vi "DAQ.vi"(0 "Queues":T1, 3 "error in (no error)":errorcluster) -> (10 "error out":errorcluster)   [LabVIEW 2014]
uses:
  CMD UI enum.ctl
  CMD Report enum.ctl
  CMD DA enum.ctl
  CMD DAQ enum.ctl
  CMD LOG enum.ctl
  set_get.ctl
  patiant and daq params.ctl
  <vilib>/DAQmx/create/channels.llb/DAQmx Create Channel (AI-Voltage-Basic).vi
  <vilib>/DAQmx/configure/timing.llb/DAQmx Timing (Sample Clock).vi
  <vilib>/DAQmx/read.llb/DAQmx Read (Analog 2D DBL NChan NSamp).vi
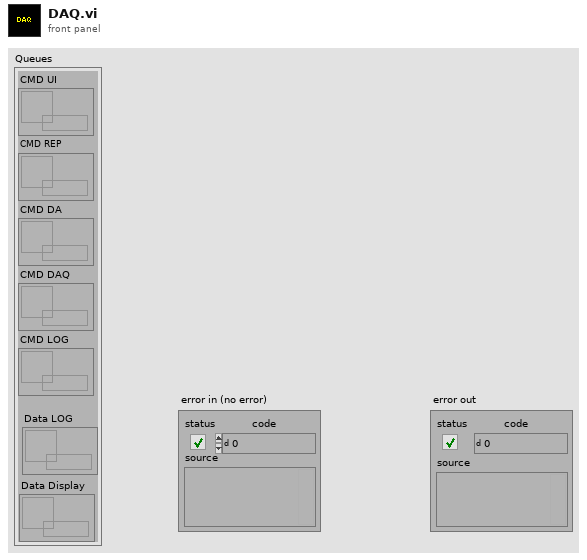
[diagram p1: front panel]
types:
  T1 = cluster{"CMD UI":refnum<queue>, "CMD REP":refnum<queue>, "CMD DA":refnum<queue>, "CMD DAQ":refnum<queue>, "CMD LOG":refnum<queue>, "Data LOG":refnum<queue>, "Data Display":refnum<queue>}
  T2 = typedef "patiant and daq params.ctl" = cluster{"DAQ Parameters":cluster{"Sampling rate":dbl, "Max_volt":dbl, "Min_volt":dbl, "DAQmx Physical Channels \nHR,SC":tag, "Resting State":bool, "Analyze every (s)":dbl}, "Patient Info \n(Updates automatically when reading from file)":cluster{"Patient Name":string, "Patient ID":string, "Patient Age":dbl, "Gender":string}, "Raw Data Read Path":path, "Avg HR ":dbl, "Avg SC  ":dbl}
  T3 = typedef "CMD DAQ enum.ctl" = enum16{"Init DAQ", "Init Read From File", "DAQ", "Read From File", "Stop DAQ", "Stop Read From File", "Exit"}
  T4 = typedef "set_get.ctl" = enum16{"Set", "Get"}
  T5 = typedef "CMD UI enum.ctl" = enum16{"Init all", "Update Patient Info", "Update Analyzed", "Create Report", "Analyze Data", "Start DAQ", "Start Read", "LOG Data", "Stop LOG Data", "Stop DAQ", "Stop Read", "EXIT"}
  T6 = enum16{"open", "replace", "create", "open or create", "replace or create", "replace or create with confirmation"}
  T7 = cluster{string, string, dbl, "Combo Box":string, dbl}
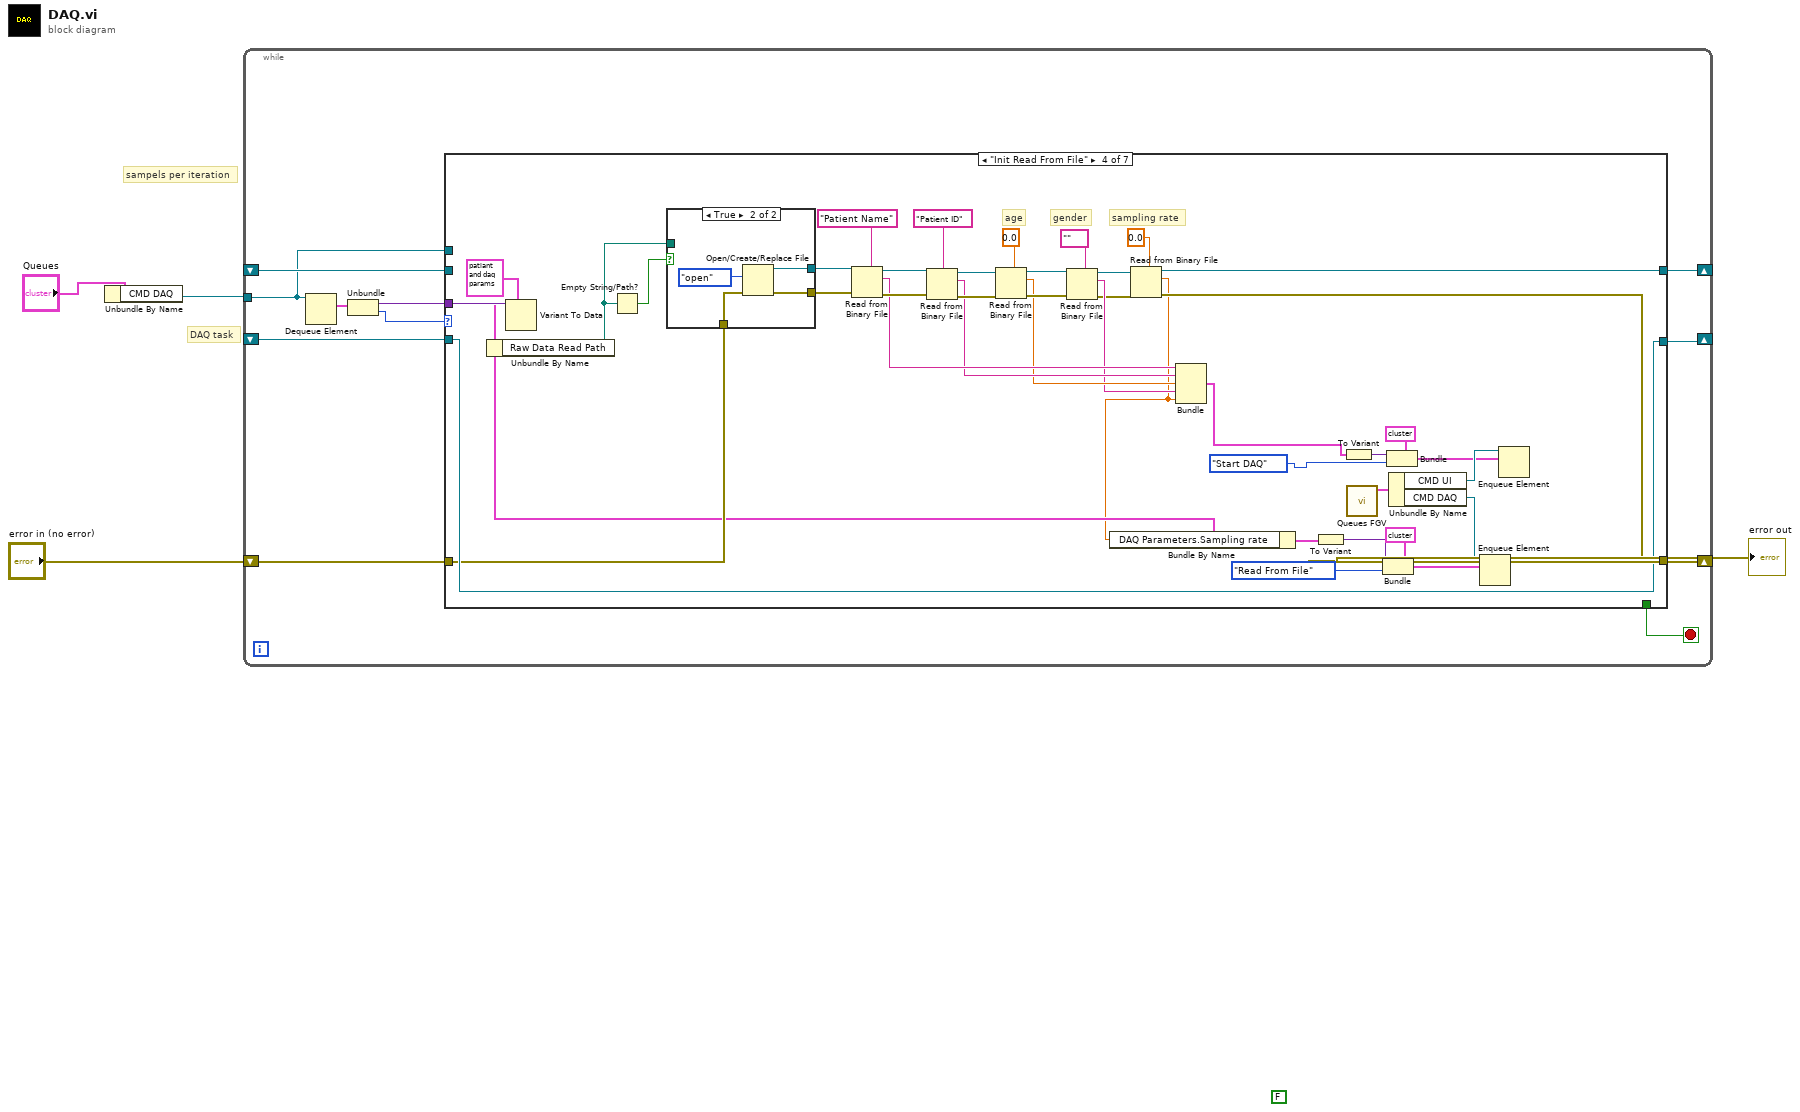
[diagram p0: block diagram]
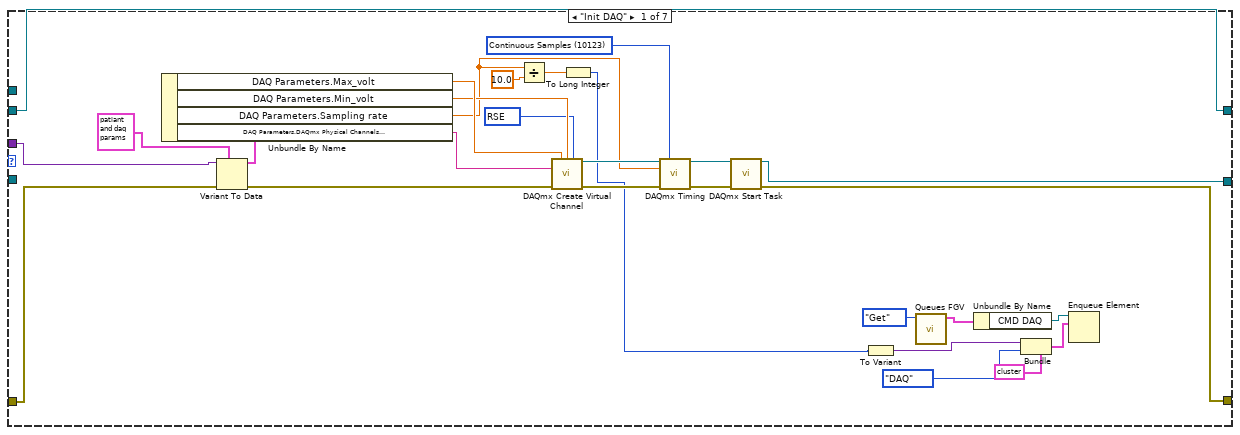
[diagram p2: hidden frame]
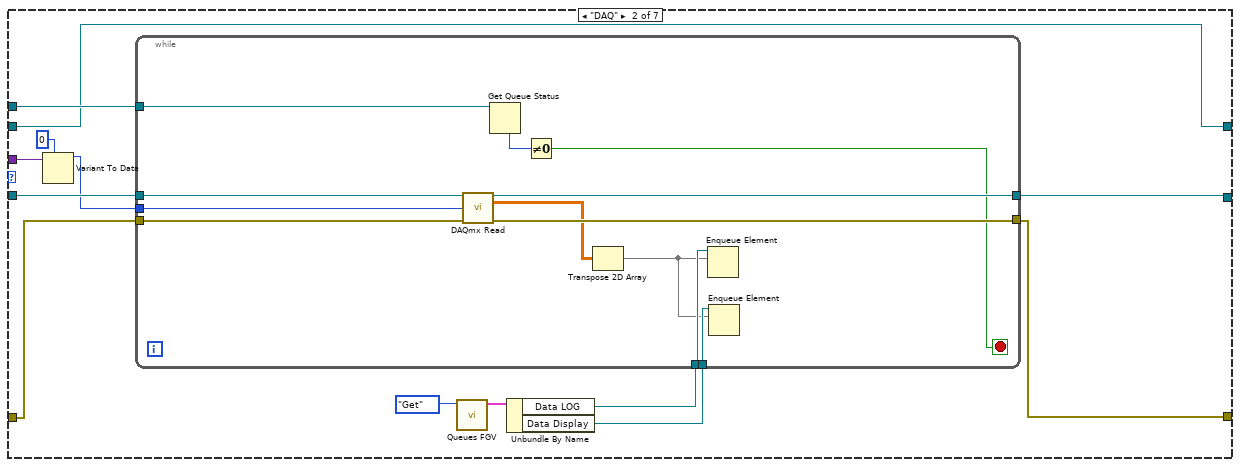
[diagram p3: hidden frame]
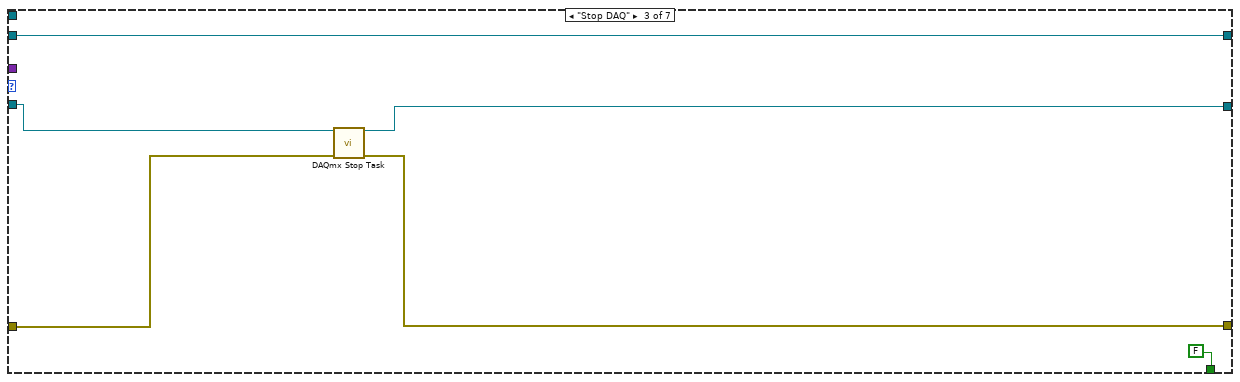
[diagram p4: hidden frame]
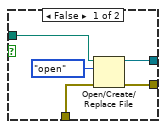
[diagram p5: hidden frame]
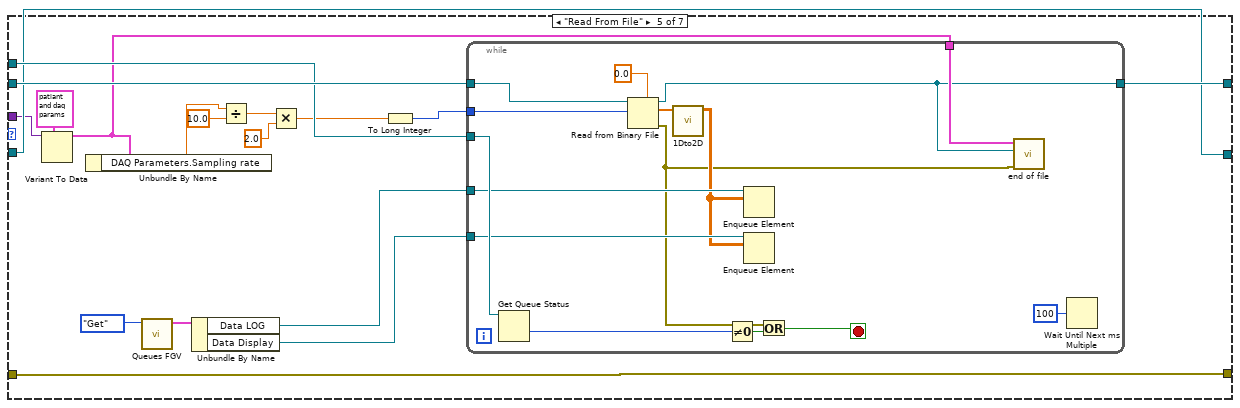
[diagram p6: hidden frame]
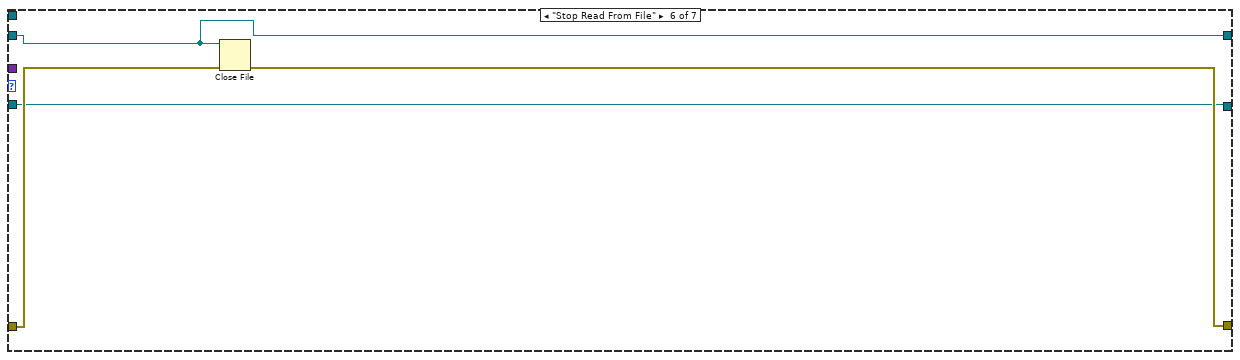
[diagram p7: hidden frame]
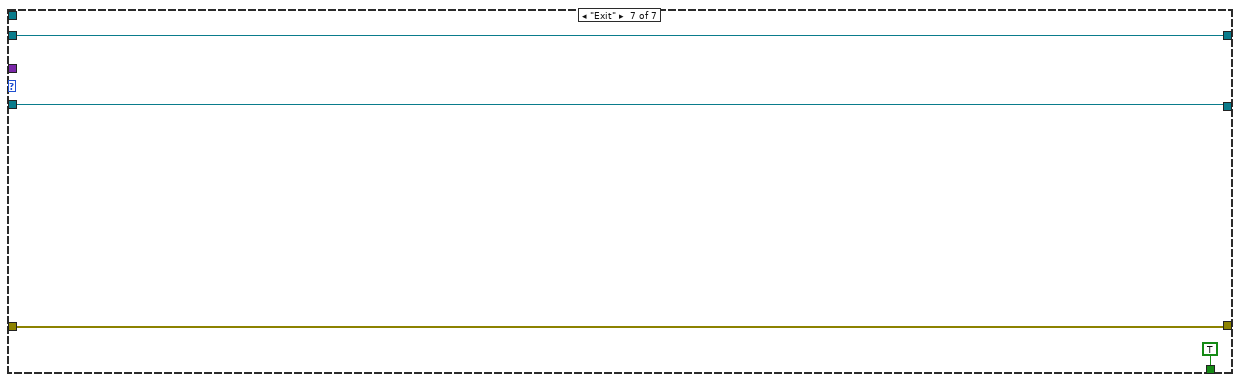
[diagram p8: hidden frame]
diagram:
  (unwired) FALSE
  # "DAQ task"
  # "sampels per iteration"
  n1 = Unbundle By Name("Queues") -> ("CMD DAQ"=w4:refnum<queue>)
  n2 = while {
    tunnel: w4 -> [w5]
    shift-right: [w12] -> w3
    shift-left: "error in (no error)" -> [w13]
    shift-right: [w10] -> _
    shift-left: _ -> [w9]
    shift-right: [w7] -> _
    shift-left: _ -> [w6]
    stop <- w11 stop-if-true
    n3 = Dequeue Element(queue=w5) -> (element=w15:cluster{variant, T3})  [unwired: 2 in, 3 out]
    n4 = Unbundle(w15) -> (w8:variant, w14:T3)
    n5 = case shown="\"Init Read From File\"" w14 {
      tunnel: [_ _ FALSE ("Boolean 2") _ _ _ TRUE ("Boolean 2")] -> w11
      tunnel: w13 -> [w31 w55 w74 w93 w136 w161 w163]
      tunnel: [w27 w54 w73 w92 w136 w160 w163] -> w12
      tunnel: [w26 w53 w72 w116 w135 w159 w165] -> w10
      tunnel: w9 -> [_ w56 w70 w116 w135 w159 w165]
      tunnel: w8 -> [w29 w48 _ w115 w127 _ _]
      tunnel: [w17 w49 w69 w94 w142 w162 w166] -> w7
      tunnel: w6 -> [w17 w49 w69 _ w143 w162 w166]
      tunnel: w5 -> [_ w50 _ _ w141 _ _]
      frame "Init DAQ" {
        w36 = 10083 items=["default"=-1, "RSE"=10083, "NRSE"=10078, "Differential"=10106, "Pseudodifferential"=12529] ("input terminal configuration")
        w41 = 10123 items=["Finite Samples"=10178, "Continuous Samples"=10123, "Hardware Timed Single Point"=12522] ("sample mode")
        n6 = Variant To Data(error in=w31, type=T2 {"DAQ Parameters"={"Sampling rate"=0.0, "Max_volt"=0.0, "Min_volt"=0.0, "DAQmx Physical Channels \nHR,SC"="", "Resting State"=FALSE, "Analyze every (s)"=0.01}, "Patient Info \n(Updates automatically when reading from file)"={"Patient Name"="", "Patient ID"="", "Patient Age"=0.0, "Gender"=""}, "Raw Data Read Path"=path "", "Avg HR "=0.0, "Avg SC  "=0.0} ("output cluster"), Variant=w29) -> (data=w40:T2, error out=w30:errorcluster)
        n7 = Unbundle By Name(w40) -> ("DAQ Parameters.Max_volt"=w38:dbl, "DAQ Parameters.Min_volt"=w37:dbl, "DAQ Parameters.Sampling rate"=w28:dbl, "DAQ Parameters.DAQmx Physical Channels \nHR,SC"=w39:tag)
        n8 = Divide(x=w28, y=10.0) -> (x/y=w32:dbl)
        n9 = call-poly <vilib>:"DAQmx Create Virtual Channel.vi"("maximum value"=w38, "minimum value"=w37, "input terminal configuration"=w36, "physical channels"=w39, "error in"=w30) -> ("task out"=w43:refnum<k21>, "error out"=w42:errorcluster)  [unwired: 9 in]
        n10 = To Long Integer(number=w32) -> (32bit integer=w18:i32)
        n11 = call-poly <vilib>:"DAQmx Timing.vi"("task/channels in"=w43, "sample mode"=w41, "rate"=w28, "error in"=w42) -> ("task out"=w35:refnum<k21>, "error out"=w34:errorcluster)  [unwired: 10 in]
        n12 = call <vilib>:"DAQmx Start Task.vi"("task/channels in"=w35, "error in"=w34) -> ("task out"=w26:refnum<k21>, "error out"=w27:errorcluster)  [unwired: 12 in]
        n13 = To Variant(anything=w18) -> (Variant=w19:variant)
        n14 = call "Queues FGV.vi"("Enum"=set_get."Get") -> ("Queues"=w21:T1)  [unwired: 10 in]
        n15 = Unbundle By Name(w21) -> ("CMD DAQ"=w22:refnum<queue>)
        n16 = Bundle(cluster=cluster{variant, T3} {variant, enum."Init DAQ"}, w19, CMD_DAQ_enum."DAQ") -> (w25:cluster{variant, T3})
        n17 = Enqueue Element(queue=w22, element=w25) -> ()  [unwired: 2 in, 3 out]
      }
      frame "DAQ" {
        n18 = Variant To Data(type=0, Variant=w48) -> (data=w46:i32)  [unwired: 1 in, 1 out]
        n19 = call "Queues FGV.vi"("Enum"=set_get."Get") -> ("Queues"=w51:T1)  [unwired: 10 in]
        n20 = Unbundle By Name(w51) -> ("Data LOG"=w45:refnum<queue>, "Data Display"=w44:refnum<queue>)
        n21 = while {
          tunnel: [w68] -> w54
          tunnel: [w67] -> w53
          tunnel: w56 -> [w66]
          tunnel: w55 -> [w65]
          tunnel: w50 -> [w62]
          tunnel: w46 -> [w61]
          tunnel: w45 -> [w60]
          tunnel: w44 -> [w59]
          stop <- w63 stop-if-true
          n22 = call-poly <vilib>:"DAQmx Read.vi"("task/channels in"=w66, "number of samples per channel"=w61, "error in"=w65) -> ("task out"=w67:refnum<k21>, "data"=w58:dbl[][], "error out"=w68:errorcluster)  [unwired: 10 in]
          n23 = Get Queue Status(queue=w62) -> (# elements in queue=w64:i32)  [unwired: 2 in, 7 out]
          n24 = Not Equal To 0?(x=w64) -> (x != 0?=w63:bool)
          n25 = Transpose 2D Array(2D array=w58) -> (transposed array=w57:dbl[][])
          n26 = Enqueue Element(queue=w60, element=w57) -> ()  [unwired: 2 in, 3 out]
          n27 = Enqueue Element(queue=w59, element=w57) -> ()  [unwired: 2 in, 3 out]
        }
      }
      frame "Stop DAQ" {
        n28 = call <vilib>:"DAQmx Stop Task.vi"("task/channels in"=w70, "error in"=w74) -> ("task out"=w72:refnum<k21>, "error out"=w73:errorcluster)  [unwired: 12 in]
      }
      frame "Init Read From File" {
        # "age"
        # "gender"
        # "sampling rate"
        n29 = Variant To Data(type=T2 {"DAQ Parameters"={"Sampling rate"=0.0, "Max_volt"=0.0, "Min_volt"=0.0, "DAQmx Physical Channels \nHR,SC"="", "Resting State"=FALSE, "Analyze every (s)"=0.01}, "Patient Info \n(Updates automatically when reading from file)"={"Patient Name"="", "Patient ID"="", "Patient Age"=0.0, "Gender"=""}, "Raw Data Read Path"=path "", "Avg HR "=0.0, "Avg SC  "=0.0} ("output cluster"), Variant=w115) -> (data=w79:T2)  [unwired: 1 in, 1 out]
        n30 = Unbundle By Name(w79) -> ("Raw Data Read Path"=w80:path)
        n31 = Empty String/Path?(string/path=w80) -> (empty?=w114:bool)
        n32 = case shown="True" w114 {
          tunnel: w80 -> [w120 _]
          tunnel: [w119 w124] -> w113
          tunnel: [w118 w123] -> w112
          tunnel: w93 -> [w117 w122]
          frame False {
            n33 = Open/Create/Replace File(file path (use dialog)=w120, error in=w117, operation (0:open)=T6."open") -> (refnum out=w119:refnum<file>, error out=w118:errorcluster)  [unwired: 3 in, 1 out]
          }
          frame True {
            n34 = Open/Create/Replace File(error in=w122, operation (0:open)=T6."open") -> (refnum out=w124:refnum<file>, error out=w123:errorcluster)  [unwired: 4 in, 1 out]
          }
        }
        n35 = Read from Binary File(5:"Patient Name", 8:w112, 11:w113) -> (0:w110:errorcluster, 2:w102:string, 3:w109:refnum<file>)  [unwired: 3 in, 1 out]
        n36 = Read from Binary File(5:"Patient ID", 8:w110, 11:w109) -> (0:w108:errorcluster, 2:w101:string, 3:w106:refnum<file>)  [unwired: 3 in, 1 out]
        n37 = Read from Binary File(5:0.0, 8:w108, 11:w106) -> (0:w107:errorcluster, 2:w100:dbl, 3:w105:refnum<file>)  [unwired: 3 in, 1 out]
        n38 = Read from Binary File(5:"" ("Combo Box"), 8:w107, 11:w105) -> (0:w97:errorcluster, 2:w99:string, 3:w96:refnum<file>)  [unwired: 3 in, 1 out]
        n39 = Read from Binary File(5:0.0, 8:w97, 11:w96) -> (0:w92:errorcluster, 2:w77:dbl, 3:w94:refnum<file>)  [unwired: 3 in, 1 out]
        n40 = Bundle By Name(cluster=w79, "DAQ Parameters.Sampling rate"=w77) -> (w78:T2)
        n41 = Bundle(w102, w101, w100, "Combo Box"=w99, w77) -> (w75:T7)  [unwired: 1 in]
        n42 = To Variant(anything=w78) -> (Variant=w87:variant)
        n43 = To Variant(anything=w75) -> (Variant=w85:variant)
        n44 = call "Queues FGV.vi"() -> ("Queues"=w98:T1)  [unwired: 11 in]
        n45 = Bundle(cluster=cluster{variant, T3} {variant, enum."Init DAQ"}, w87, CMD_DAQ_enum."Read From File") -> (w88:cluster{variant, T3})
        n46 = Bundle(cluster=cluster{variant, T5} {variant, enum."Start DAQ"}, w85, CMD_UI_enum."Start DAQ") -> (w82:cluster{variant, T5})
        n47 = Unbundle By Name(w98) -> ("CMD UI"=w84:refnum<queue>, "CMD DAQ"=w91:refnum<queue>)
        n48 = Enqueue Element(queue=w91, element=w88) -> ()  [unwired: 2 in, 3 out]
        n49 = Enqueue Element(queue=w84, element=w82) -> ()  [unwired: 2 in, 3 out]
      }
      frame "Read From File" {
        n50 = Variant To Data(type=T2 {"DAQ Parameters"={"Sampling rate"=0.0, "Max_volt"=0.0, "Min_volt"=0.0, "DAQmx Physical Channels \nHR,SC"="", "Resting State"=FALSE, "Analyze every (s)"=0.01}, "Patient Info \n(Updates automatically when reading from file)"={"Patient Name"="", "Patient ID"="", "Patient Age"=0.0, "Gender"=""}, "Raw Data Read Path"=path "", "Avg HR "=0.0, "Avg SC  "=0.0} ("output cluster"), Variant=w127) -> (data=w126:T2)  [unwired: 1 in, 1 out]
        n51 = Unbundle By Name(w126) -> ("DAQ Parameters.Sampling rate"=w128:dbl)
        n52 = call "Queues FGV.vi"("Enum"=set_get."Get") -> ("Queues"=w140:T1)  [unwired: 10 in]
        n53 = Unbundle By Name(w140) -> ("Data LOG"=w138:refnum<queue>, "Data Display"=w137:refnum<queue>)
        n54 = Divide(x=w128, y=10.0) -> (x/y=w133:dbl)
        n55 = Multiply(x=w133, y=2.0) -> (x*y=w131:dbl)
        n56 = To Long Integer(number=w131) -> (32bit integer=w130:i32)
        n57 = while {
          tunnel: w143 -> [w158]
          tunnel: [w145] -> w142
          tunnel: w141 -> [w156]
          tunnel: w138 -> [w155]
          tunnel: w137 -> [w154]
          tunnel: w130 -> [w147]
          tunnel: w126 -> [w146]
          stop <- w148 stop-if-true
          n58 = Get Queue Status(queue=w156) -> (# elements in queue=w157:i32)  [unwired: 2 in, 7 out]
          n59 = Read from Binary File(5:0.0, 10:w147, 11:w158) -> (0:w144:errorcluster, 2:w151:dbl[], 3:w145:refnum<file>)  [unwired: 3 in, 1 out]
          n60 = call "1Dto2D.vi"("Array"=w151) -> ("output array"=w150:dbl[][])  [unwired: 10 in]
          n61 = Not Equal To 0?(x=w157) -> (x != 0?=w149:bool)
          n62 = Enqueue Element(queue=w155, element=w150) -> ()  [unwired: 2 in, 3 out]
          n63 = Enqueue Element(queue=w154, element=w150) -> ()  [unwired: 2 in, 3 out]
          n64 = Or(x=w144, y=w149) -> (x .or. y?=w148:bool)
          n65 = call "end of file.vi"("error in (no error)"=w144, "refnum out"=w145, "output cluster"=w146) -> ()  [unwired: 8 in, 1 out]
          n66 = Wait Until Next ms Multiple(millisecond multiple=u32 100) -> ()  [unwired: 1 out]
        }
      }
      frame "Stop Read From File" {
        n67 = Close File(refnum=w162, error in=w161) -> (error out=w160:errorcluster)  [unwired: 1 out]
      }
      frame "Exit" {
      }
    }
  }
  "error out" <- w3
